vi "U8ToSTR.vi"(4 "Index":u32, 5 "Count":i32=1, 7 "Input U8 Array":u8[](array[numeric])) -> (0 "Index+Count":u32, 1 "Output String":string, 3 "Output U8 Array":u8[](array[numeric]))   [LabVIEW 2017]
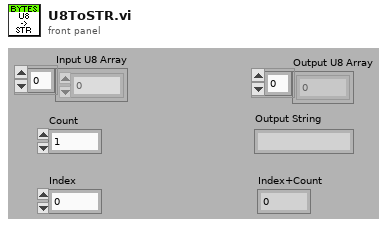
[diagram p1: front panel]
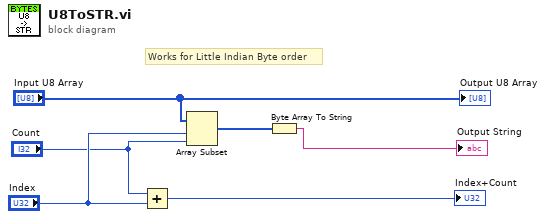
[diagram p0: block diagram]
diagram:
  # "Works for Little Indian Byte order"
  n1 = Add(x="Count", y="Index") -> (x+y=→"Index+Count":u32)
  n2 = Array Subset(array="Input U8 Array", index="Index", length="Count") -> (w3:u8[])
  n3 = Byte Array To String(unsigned byte array=w3) -> (string=→"Output String":string)
  "Output U8 Array" <- "Input U8 Array"
